vi "HardwarePresent.vi"() -> ()   [LabVIEW 2013]
panel:
  in  "HardwarePresent":bool
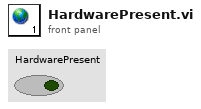
[diagram p1: front panel]
diagram:
